vi "TAV_Query.vi"(0 "System no.":i32=1 min=1 max=4 step=1, 1 "Board":i32=1 min=1 max=10 step=1, 2 "Query":u16(ring) items=["Value", "Range", "Power unit"], 5 "error in":errorcluster) -> (14 "Analog value":dbl format="%.6f", 15 "Range":dbl min=0.0 max=1.0 step=1.0, 16 "Power unit":string, 19 "error out":errorcluster)   [LabVIEW 2020]
doc: "Returns the current analog value in volts, the range of the optical head or the power unit of the Analog value, depending on \"Query\". Query time for Analog value will depend on \"NAV\" settings.\n\nC-865, C-866: Query = Value, Board = 1. Range and Power unit are not valid.\n\nC-867, C-884, E-861, E-871, E-873, E-874, Mercury_GCS: Query = Value, Board = 1 to 4. Range and Power unit are not valid. \n\nC-880: Query = Value. Range and Power unit are not valid\n\nE-712, E-727: \nE-761: Query = Value, Board = 4. Range and Power unit are not valid. The output is the current voltage at the analog input line, with gain and offset.\n\nC-887, F-206, M-8X0: For GCS syntax version = GCS 1.0 (check with CSV?.vi. If CSV?.vi is not supported, syntax version is GCS 1.0), Query can be Value, Range or Power unit. For GCS syntax version = GCS 2.0 or higher, Query = Value \n\nMercury: Query = Value. Board = analog input channel ID, can be 1-4, 5-7, 8-11 etc., see GCS DLL Manual for details. Range and Power unit are not valid"
uses:
  Global1.vi
panel:
  # "Returns the current analog value in volts, range or power unit, depending on \"Query\". Query time for Analog value will depend on NAV settings."
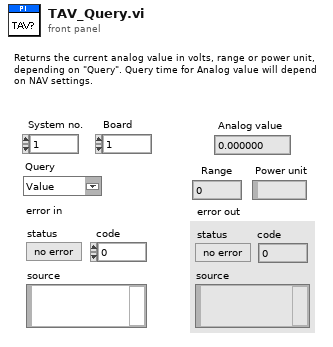
[diagram p1: front panel]
types:
  T1 = typedef "Syntax.ctl" = enum16{"GCS 1.0", "GCS 2.0", "GCS 3.0"}
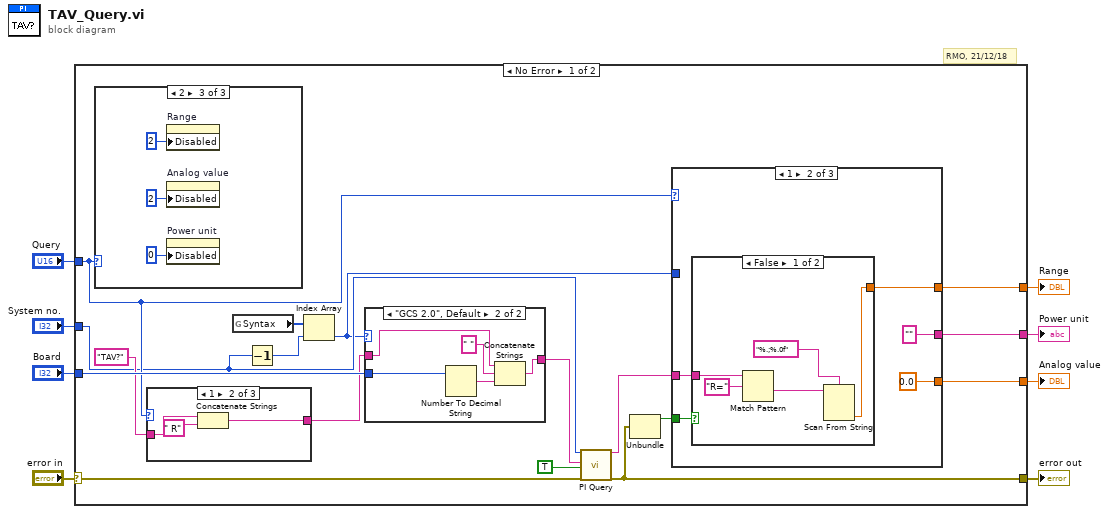
[diagram p0: block diagram]
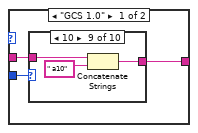
[diagram p2: hidden frame]
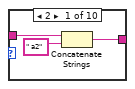
[diagram p3: hidden frame]
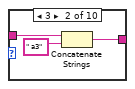
[diagram p4: hidden frame]
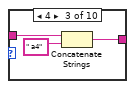
[diagram p5: hidden frame]
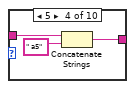
[diagram p6: hidden frame]
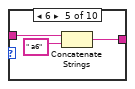
[diagram p7: hidden frame]
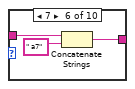
[diagram p8: hidden frame]
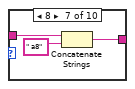
[diagram p9: hidden frame]
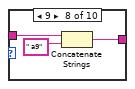
[diagram p10: hidden frame]
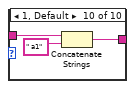
[diagram p11: hidden frame]
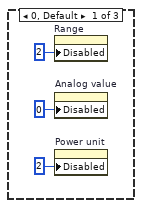
[diagram p12: hidden frame]
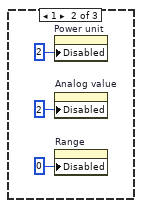
[diagram p13: hidden frame]
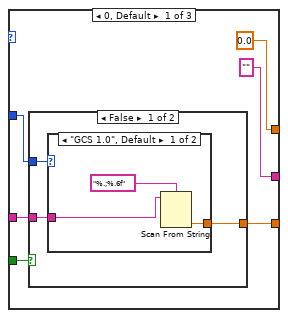
[diagram p14: hidden frame]
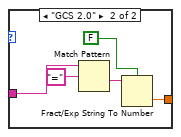
[diagram p15: hidden frame]
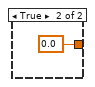
[diagram p16: hidden frame]
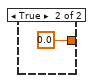
[diagram p17: hidden frame]
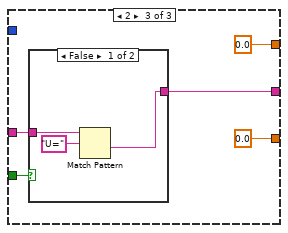
[diagram p18: hidden frame]
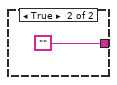
[diagram p19: hidden frame]
diagram:
  # "RMO, 21/12/18"
  n1 = case shown="No Error" "error in" {
    selector: "error in" -> [w11 w120]
    tunnel: [w10 w120] -> w8
    tunnel: "Board" -> [w24 _]
    tunnel: "Query" -> [w19 _]
    tunnel: "System no." -> [w17 _]
    tunnel: [w14 w119] -> w4
    tunnel: [w13 w119] -> w3
    tunnel: [w12 "" ("String read")] -> w2
    frame No Error {
      n2 = case shown="2" w19 {
        frame 0, Default {
          n3 = property on="Range" class="DigNum (strict)"("Disabled"=u8 2) -> ()  [unwired: 2 in, 2 out]
          n4 = property on="Analog value" class="DigNum (strict)"("Disabled"=u8 0) -> ()  [unwired: 2 in, 2 out]
          n5 = property on="Power unit" class="Str"("Disabled"=u8 2) -> ()  [unwired: 2 in, 2 out]
        }
        frame 1 {
          n6 = property on="Power unit" class="Str"("Disabled"=u8 2) -> ()  [unwired: 2 in, 2 out]
          n7 = property on="Analog value" class="DigNum (strict)"("Disabled"=u8 2) -> ()  [unwired: 2 in, 2 out]
          n8 = property on="Range" class="DigNum (strict)"("Disabled"=u8 0) -> ()  [unwired: 2 in, 2 out]
        }
        frame 2 {
          n9 = property on="Range" class="DigNum (strict)"("Disabled"=u8 2) -> ()  [unwired: 2 in, 2 out]
          n10 = property on="Analog value" class="DigNum (strict)"("Disabled"=u8 2) -> ()  [unwired: 2 in, 2 out]
          n11 = property on="Power unit" class="Str"("Disabled"=u8 0) -> ()  [unwired: 2 in, 2 out]
        }
      }
      n12 = case shown="1" w19 {
        tunnel: "TAV?" -> [w111 w113 w116]
        tunnel: [w111 w112 w115] -> w21
        frame 0, Default {
        }
        frame 1 {
          n13 = Concatenate Strings(w113, " R" ("Substring")) -> (w112:string)
        }
        frame 2 {
          n14 = Concatenate Strings(w116, " U" ("Substring")) -> (w115:string)
        }
      }
      n15 = global read "Global1.vi" "Syntax"() -> (w18:T1[])
      n16 = Decrement(x=w17) -> (x-1=w16:i32)
      n17 = Index Array(array=w18, index=w16) -> (element=w15:T1)
      n18 = case shown="\"GCS 2.0\", Default" w15 {
        tunnel: w24 -> [w28 w63]
        tunnel: [w27 w61] -> w23
        tunnel: w21 -> [w26 w62]
        frame "GCS 1.0" {
          n19 = case shown="10" w28 {
            tunnel: w26 -> [w31 w34 w37 w40 w43 w46 w49 w52 w55 w58]
            tunnel: [w29 w32 w35 w38 w41 w44 w47 w50 w53 w56] -> w27
            frame 2 {
              n20 = Concatenate Strings(w31, " a2" ("Substring")) -> (w29:string)
            }
            frame 3 {
              n21 = Concatenate Strings(w34, " a3" ("Substring")) -> (w32:string)
            }
            frame 4 {
              n22 = Concatenate Strings(w37, " a4" ("Substring")) -> (w35:string)
            }
            frame 5 {
              n23 = Concatenate Strings(w40, " a5" ("Substring")) -> (w38:string)
            }
            frame 6 {
              n24 = Concatenate Strings(w43, " a6" ("Substring")) -> (w41:string)
            }
            frame 7 {
              n25 = Concatenate Strings(w46, " a7" ("Substring")) -> (w44:string)
            }
            frame 8 {
              n26 = Concatenate Strings(w49, " a8" ("Substring")) -> (w47:string)
            }
            frame 9 {
              n27 = Concatenate Strings(w52, " a9" ("Substring")) -> (w50:string)
            }
            frame 10 {
              n28 = Concatenate Strings(w55, " a10" ("Substring")) -> (w53:string)
            }
            frame 1, Default {
              n29 = Concatenate Strings(w58, " a1" ("Substring")) -> (w56:string)
            }
          }
        }
        frame "GCS 2.0", Default {
          n30 = Number To Decimal String(number=w63) -> (decimal integer string=w60:string)  [unwired: 1 out]
          n31 = Concatenate Strings(w62, " " ("string"), w60) -> (w61:string)
        }
      }
      n32 = call "PI Query.vi"("System no."=w17, "String to send"=w23, "Attach termination char.?"=TRUE ("Attach Linefeed?"), "error in"=w11) -> ("String read"=w9:string, "error out"=w10:errorcluster)  [unwired: 3 in, 11 out]
      n33 = Unbundle(w10) -> ("status"=w20:bool)  [unwired: 2 out]
      n34 = case shown="1" w19 {
        tunnel: w20 -> [w78 w95 w106]
        tunnel: w9 -> [w77 w94 w105]
        tunnel: w15 -> [w76 _ _]
        tunnel: [w75 0.0 0.0] -> w14
        tunnel: [0.0 w93 0.0] -> w13
        tunnel: ["" ("String read") "" ("String read") w104] -> w12
        frame 0, Default {
          n35 = case shown="False" w78 {
            tunnel: w77 -> [w81 _]
            tunnel: [w80 0.0] -> w75
            tunnel: w76 -> [w79 _]
            frame False {
              n36 = case shown="\"GCS 1.0\", Default" w79 {
                tunnel: w81 -> [w84 w89]
                tunnel: [w82 w86] -> w80
                frame "GCS 1.0", Default {
                  n37 = Scan From String(format string="%.;%.6f" ("Format String"), input string=w84) -> (output 1=w82:dbl)  [unwired: 2 in, 4 out]
                }
                frame "GCS 2.0" {
                  n38 = Match Pattern(string=w89, regular expression="=") -> (after substring=w87:string)  [unwired: 4 out]
                  n39 = Fract/Exp String To Number(use system decimal point (T)=FALSE, string=w87) -> (number=w86:dbl)  [unwired: 3 out]
                }
              }
            }
            frame True {
            }
          }
        }
        frame 1 {
          n40 = case shown="False" w95 {
            tunnel: w94 -> [w97 _]
            tunnel: [w99 0.0] -> w93
            frame False {
              n41 = Match Pattern(string=w97, regular expression="R=") -> (after substring=w96:string)  [unwired: 4 out]
              n42 = Scan From String(format string="%.;%.0f" ("Format String"), input string=w96) -> (output 1=w99:dbl)  [unwired: 2 in, 4 out]
            }
            frame True {
            }
          }
        }
        frame 2 {
          n43 = case shown="False" w106 {
            tunnel: w105 -> [w108 _]
            tunnel: [w107 ""] -> w104
            frame False {
              n44 = Match Pattern(string=w108, regular expression="U=") -> (after substring=w107:string)  [unwired: 4 out]
            }
            frame True {
            }
          }
        }
      }
    }
    frame Error {
      w119 = 0.0
    }
  }
  "error out" <- w8
  "Analog value" <- w4
  "Range" <- w3
  "Power unit" <- w2
